vi "Compare Head to Tail Distance (SubVI).vi"(7 "Min Distance":i16=1600, 11 "HT-LOC":u64) -> (3 "Valid?":bool)   [LabVIEW 2015]
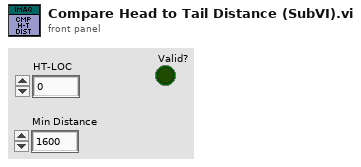
[diagram p1: front panel]
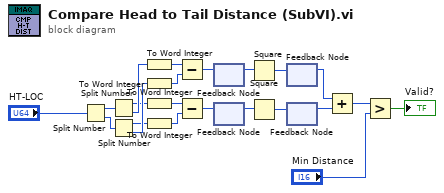
[diagram p0: block diagram]
diagram:
  n1 = Split Number(x="HT-LOC") -> (hi(x)=w1:u32, lo(x)=w2:u32)
  n2 = Split Number(x=w1) -> (hi(x)=w3:u16, lo(x)=w5:u16)
  n3 = Split Number(x=w2) -> (hi(x)=w4:u16, lo(x)=w6:u16)
  n4 = To Word Integer(number=w5) -> (16bit integer=w12:i16)
  n5 = To Word Integer(number=w6) -> (16bit integer=w14:i16)
  n6 = To Word Integer(number=w3) -> (16bit integer=w11:i16)
  n7 = To Word Integer(number=w4) -> (16bit integer=w13:i16)
  n8 = Subtract(x=w12, y=w14) -> (x-y=w8:i16)
  n9 = Subtract(x=w11, y=w13) -> (x-y=w7:i16)
  n10 = feedback #1() -> (w19:i16)  [unwired: 1 in]
  n11 = feedback-in #1(w8) -> ()
  n12 = feedback #2() -> (w18:i16)  [unwired: 1 in]
  n13 = feedback-in #2(w7) -> ()
  n14 = Square(x=w19) -> (x^2=w10:i16)
  n15 = Square(x=w18) -> (x^2=w9:i16)
  n16 = feedback #3() -> (w21:i16)  [unwired: 1 in]
  n17 = feedback-in #3(w10) -> ()
  n18 = feedback #4() -> (w20:i16)  [unwired: 1 in]
  n19 = feedback-in #4(w9) -> ()
  n20 = Add(x=w21, y=w20) -> (x+y=w15:i16)
  n21 = Greater?(x=w15, y="Min Distance") -> (0:→"Valid?":bool)
